vi "oa_SCL Count Data Points.vi"(0 "scaled xy data":cluster{"x":i16, "y":i16}[](array[cluster])) -> (1 "counted data":cluster{"x":i16, "y":i16, "c":i16}[](array[cluster]), 2 "max count":i16)   [LabVIEW 2017]
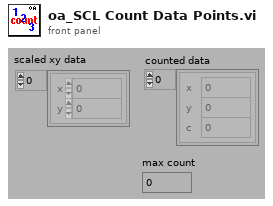
[diagram p1: front panel]
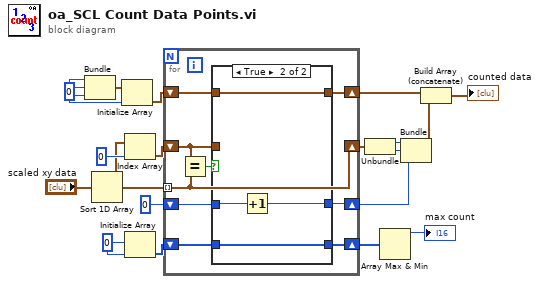
[diagram p0: block diagram]
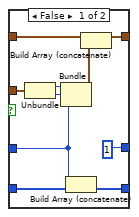
[diagram p2: hidden frame]
diagram:
  w4 = i16 0
  w14 = i16 0
  n1 = Bundle(w14, w14, w14) -> (w15:cluster{i16, i16, i16})  [unwired: 1 in]
  n2 = Sort 1D Array(array="scaled xy data") -> (sorted array=w13:cluster{"x":i16, "y":i16}[])
  n3 = Initialize Array(w15, w14) -> (w16:cluster{i16, i16, i16}[])
  n4 = Index Array(array=w13, index=0) -> (element=w17:cluster{"x":i16, "y":i16})
  n5 = Initialize Array(w4, w4) -> (w3:i16[])
  n6 = for {
    shift-right: [w22] -> w10
    shift-left: w17 -> [w23]
    shift-right: [w26] -> w9
    shift-left: i16 0 -> [w27]
    tunnel: w13 -> [w22] mode=indexing
    shift-right: [w24] -> w8
    shift-left: w16 -> [w25]
    shift-right: [w20] -> w2
    shift-left: w3 -> [w21]
    n7 = Equal?(x=w23, y=w22) -> (x = y?=w28:bool)
    n8 = case shown="True" w28 {
      tunnel: w27 -> [w29 w42]
      tunnel: [i16 1 w41] -> w26
      tunnel: w23 -> [w32 _]
      tunnel: w25 -> [w35 w40]
      tunnel: [w34 w40] -> w24
      tunnel: w21 -> [w31 w39]
      tunnel: [w30 w39] -> w20
      frame False {
        n9 = Unbundle(w32) -> ("x"=w37:i16, "y"=w36:i16)
        n10 = Bundle("x"=w37, "y"=w36, w29) -> (w33:cluster{"x":i16, "y":i16, i16})  [unwired: 1 in]
        n11 = Build Array (concatenate)(w29, w31) -> (w30:i16[])
        n12 = Build Array (concatenate)(w35, w33) -> (w34:cluster{"x":i16, "y":i16, i16}[])
      }
      frame True {
        n13 = Increment(x=w42) -> (x+1=w41:i16)
      }
    }
  }
  n14 = Unbundle(w10) -> ("x"=w11:i16, "y"=w12:i16)
  n15 = Array Max & Min(array=w2) -> (max value=→"max count":i16)  [unwired: 3 out]
  n16 = Bundle("x"=w11, "y"=w12, w9) -> (w7:cluster{"x":i16, "y":i16, i16})  [unwired: 1 in]
  n17 = Build Array (concatenate)(w8, w7) -> (→"counted data":cluster{"x":i16, "y":i16, i16}[])
